vi "Init Port.vi"(8 "error in (no error)":errorcluster, 10 "BAUD":u16, 11 "String":string) -> (0 "error out":errorcluster, 3 "VISA Refnum out":refnum<visa-resource-name>)   [LabVIEW 2020]
uses:
  <vilib>/Instr/_visa.llb/VISA Open Access Mode.ctl
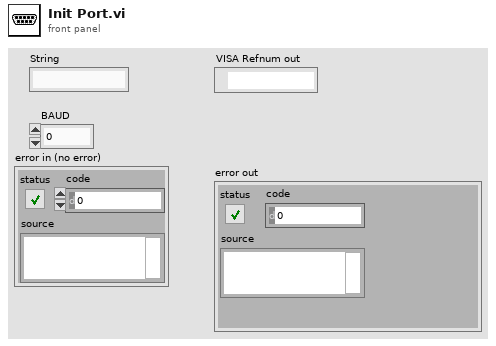
[diagram p1: front panel]
types:
  T1 = typedef "VISA Open Access Mode.ctl" = u32
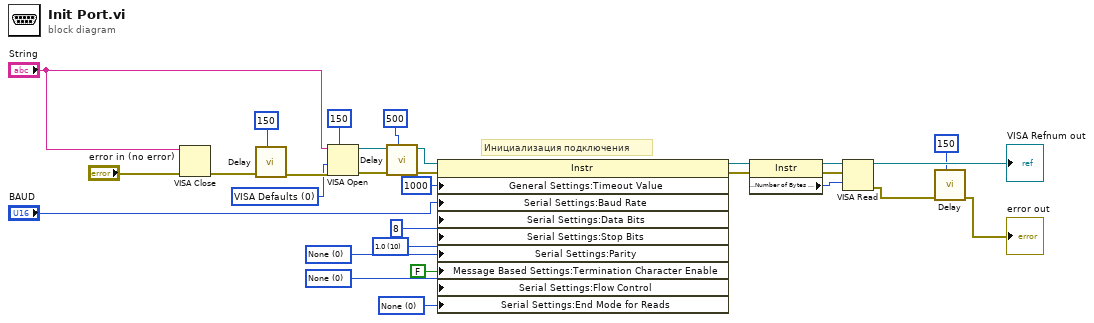
[diagram p0: block diagram]
diagram:
  w5 = T1 0 items=["VISA Defaults"=0, "Exclusive Lock"=1, "Load Configured Settings"=4] ("Access Mode")
  w29 = u16 0 items=["None", "Odd", "Even", "Mark", "Space"] ("Serial Settings:Parity")
  w27 = u16 0 items=["None", "XON/XOFF", "RTS/CTS", "XON/XOFF & RTS/CTS", "DTR/DSR", "XON/XOFF & DTR/DSR"] ("Serial Settings:Flow Control")
  w16 = u16 0 items=["None", "LastBit", "TermChar"] ("Serial Settings:Serial End Mode for Reads")
  w14 = u16 10 items=["1.0"=10, "1.5"=15, "2.0"=20] ("Serial Settings:Serial Stop Bits")
  # "Инициализация подключения"
  n1 = VISA Close(VISA resource name="String", error in (no error)="error in (no error)") -> (error out=w9:errorcluster)
  n2 = call "Delay.vi"("milliseconds to wait"=u32 150, "error in (no error)"=w9) -> ("error out"=w8:errorcluster)  [unwired: 8 in, 1 out]
  n3 = VISA Open(timeout (0)=u32 150 ("VISA Open timeout (0)"), access mode=w5, error in (no error)=w8, VISA resource name="String") -> (VISA resource name=w3:refnum<visa-resource-name>, error out=w21:errorcluster)  [unwired: 1 in]
  n4 = call "Delay.vi"("milliseconds to wait"=u32 500, "error in (no error)"=w21, "VISA Refnum  In"=w3) -> ("error out"=w22:errorcluster, "VISA Refnum out"=w2:refnum<visa-resource-name>)  [unwired: 7 in]
  n5 = property class="Instr"(reference=w2, error in=w22, "General Settings:Timeout Value"=u32 1000, "Serial Settings:Baud Rate"="BAUD", "Serial Settings:Data Bits"=u16 8 ("data bits"), "Serial Settings:Stop Bits"=w14, "Serial Settings:Parity"=w29, "Message Based Settings:Termination Character Enable"=FALSE, "Serial Settings:Flow Control"=w27, "Serial Settings:End Mode for Reads"=w16) -> (reference out=w18:refnum<visa-resource-name>, error out=w26:errorcluster)
  n6 = property class="Instr"(reference=w18, error in=w26) -> (reference out=w24:refnum<visa-resource-name>, error out=w23:errorcluster, "Serial Settings:Number of Bytes at Serial Port"=w20:u32)
  n7 = VISA Read(VISA resource name=w24, byte count=w20, error in (no error)=w23) -> (VISA resource name out=→"VISA Refnum out":refnum<visa-resource-name>, error out=w13:errorcluster)  [unwired: 2 out]
  n8 = call "Delay.vi"("milliseconds to wait"=u32 150, "error in (no error)"=w13) -> ("error out"=→"error out":errorcluster)  [unwired: 8 in, 1 out]
